vi "Execution_Message_Act.vi"(7 "EVE reference in":refnum<data-value>, 8 "error in (no error)":errorcluster, 11 "ErrorMessage in":refnum<class "ErrorMessage.lvclass">) -> (0 "error out":errorcluster, 3 "ErrorMessage out":refnum<class "ErrorMessage.lvclass">)   [LabVIEW 2013, in "ErrorMessage.lvclass"]
uses:
  ErrorMessage.lvclass
  EVE/EVE.lvclass
  Messages.lvclass
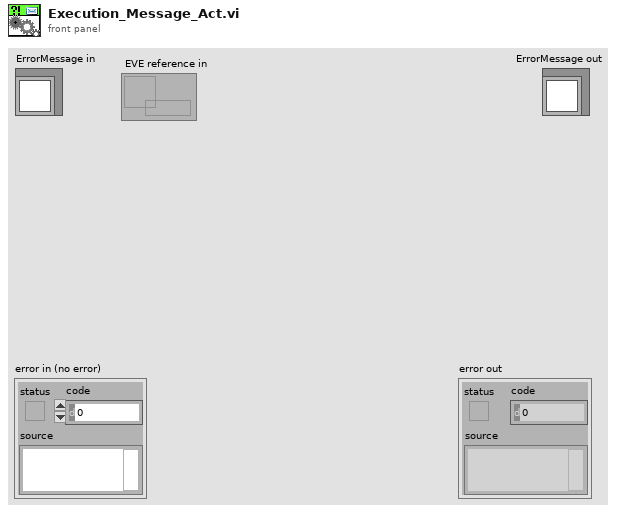
[diagram p1: front panel]
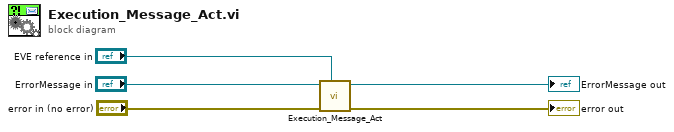
[diagram p0: block diagram]
diagram:
  n1 = call-parent "Execution_Message_Act.vi"("EVE reference in"="EVE reference in", "error in (no error)"="error in (no error)", "Messages in"="ErrorMessage in") -> ("error out"=→"error out":errorcluster, "Messages out"=→"ErrorMessage out":refnum<class "ErrorMessage.lvclass">)  [unwired: 7 in]
